vi "DDS - Sin Triangle.vi"(7 "Reset Accumulator":bool, 9 "Wave":enum16{"Triangle", "Sine", "Ramp"}(ring), 10 "Accumulator Increment":fxp<+,32,32>) -> (1 "Accumulator Value":fxp<+,32,32>, 2 "data out":i16 caption="Sine Data Out")   [LabVIEW 2015]
uses:
  <vilib>/rvi/FXPMathLib/FxpAdd/XNode/nifxpmath_Add.xnode
  <vilib>/rvi/FXPMathLib/sim/FxpSim.dll
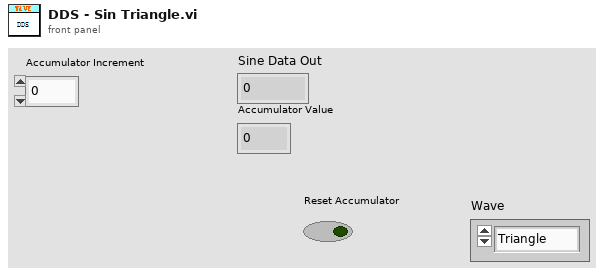
[diagram p1: front panel]
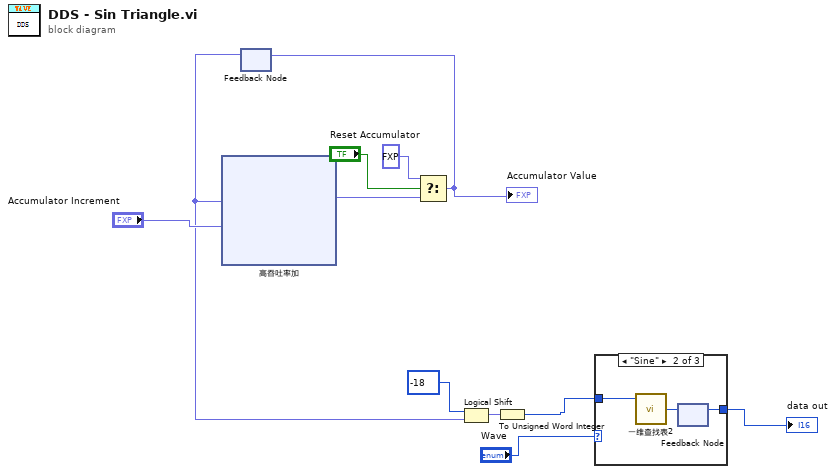
[diagram p0: block diagram]
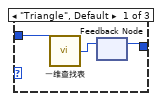
[diagram p2: hidden frame]
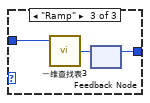
[diagram p3: hidden frame]
diagram:
  n1 = feedback #1() -> (w4:fxp<+,32,32>)  [unwired: 1 in]
  n2 = xnode ("高吞吐率加")("x"=w4, "y"="Accumulator Increment") -> ("x+y"=w9:fxp<+,32,32>)
  n3 = Select(t=fxp<+,32,32> 0.0, s="Reset Accumulator", f=w9) -> (s? t:f=w10:fxp<+,32,32>)
  "Accumulator Value" <- w10
  n4 = feedback-in #1(w10) -> ()
  n5 = Logical Shift(y=i16 -18, x=w4) -> (x << y=w5:fxp<+,32,32>)
  n6 = To Unsigned Word Integer(number=w5) -> (unsigned 16bit integer=w2:u16)
  n7 = case shown="\"Sine\"" "Wave" {
    tunnel: [w12 w15 w18] -> w1
    tunnel: w2 -> [w14 w17 w20]
    frame "Triangle", Default {
      n8 = call "一维查找表"("address"=w14) -> ("data out"=w13:i16)  [unwired: 8 in]
      n9 = feedback #2 ("反馈节点")() -> (w12:i16)  [unwired: 1 in]
      n10 = feedback-in #2(w13) -> ()
    }
    frame "Sine" {
      n11 = call "一维查找表2"("address"=w17) -> ("data out"=w16:i16)  [unwired: 8 in]
      n12 = feedback #3 ("反馈节点")() -> (w15:i16)  [unwired: 1 in]
      n13 = feedback-in #3(w16) -> ()
    }
    frame "Ramp" {
      n14 = call "一维查找表3"("address"=w20) -> ("data out"=w19:i16)  [unwired: 8 in]
      n15 = feedback #4 ("反馈节点")() -> (w18:i16)  [unwired: 1 in]
      n16 = feedback-in #4(w19) -> ()
    }
  }
  "data out" <- w1
